vi "ASIC_CONFIGURAR IABIAS.vi"(7 "Espera acceso USB":u32=10, 8 "error in":errorcluster, 9 "IBIAS VALUE":u8 max=63 step=1, 10 "IBIAS":bool, 11 "ftHandle_in":u32) -> (0 "error out":errorcluster, 3 "ftHandle_out":u32)   [LabVIEW 2019]
panel:
  out "test":u16 format="%04x"
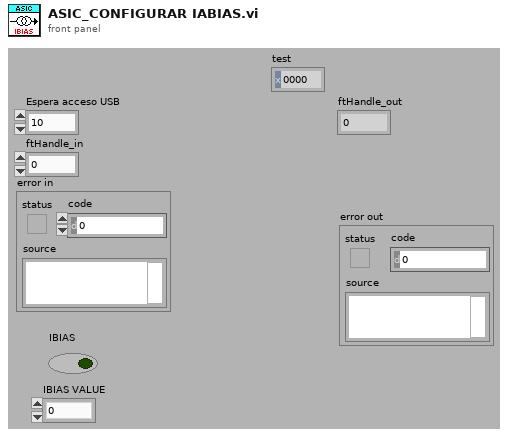
[diagram p1: front panel]
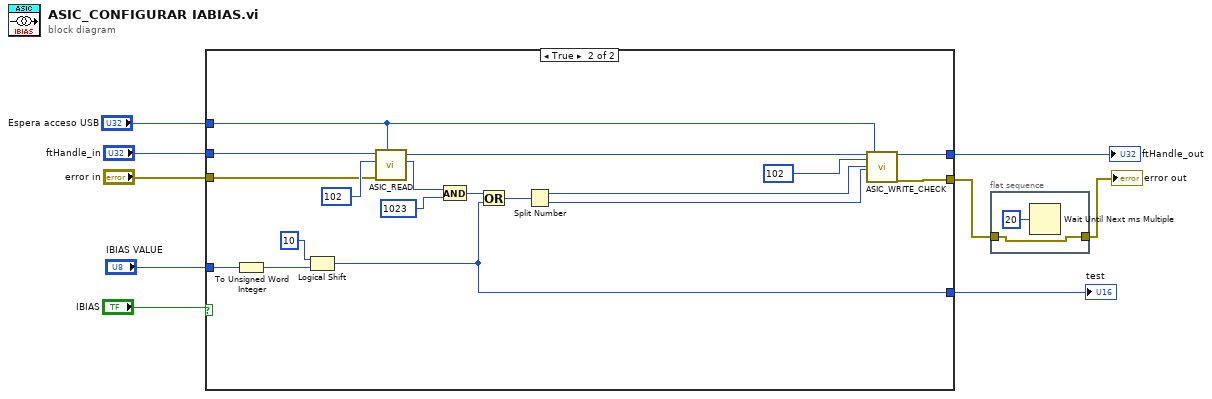
[diagram p0: block diagram]
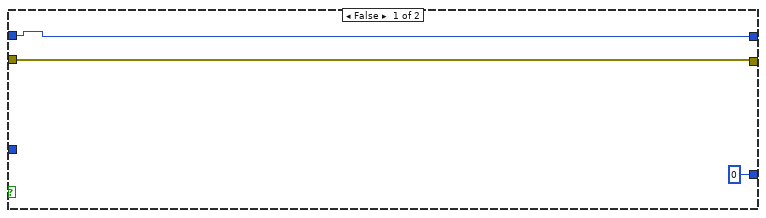
[diagram p2: hidden frame]
diagram:
  n1 = case shown="True" "IBIAS" {
    tunnel: [w10 w30] -> w9
    tunnel: [w12 w29] -> w2
    tunnel: "ftHandle_in" -> [w10 w26]
    tunnel: "error in" -> [w12 w25]
    tunnel: "Espera acceso USB" -> [_ w24]
    tunnel: [u16 0 w15] -> w5
    tunnel: "IBIAS VALUE" -> [_ w14]
    frame False {
    }
    frame True {
      n2 = To Unsigned Word Integer(number=w14) -> (unsigned 16bit integer=w13:u16)
      n3 = Logical Shift(y=u16 10 ("x"), x=w13) -> (x << y=w15:u16)
      n4 = call "ASIC_READ.vi"("Espera acceso USB"=w24, "error in"=w25, "Direccion Registro Asic"=u8 102, "ftHandle_in"=w26) -> ("Valor Asic"=w20:u16, "ftHandle_out"=w23:u32)  [unwired: 5 in, 1 out]
      n5 = And(x=w20, y=u16 1023) -> (x .and. y?=w18:u16)
      n6 = Or(x=w18, y=w15) -> (x .or. y?=w17:u16)
      n7 = Split Number(x=w17) -> (hi(x)=w22:u8, lo(x)=w21:u8)
      n8 = call "ASIC_WRITE_CHECK.vi"("ftHandle_in"=w23, "Direccion Registro Asic"=u8 102, "Byte Alto"=w22, "Byte Bajo"=w21, "Espera acceso USB 2"=w24) -> ("ftHandle_out"=w30:u32, "error out"=w29:errorcluster)  [unwired: 12 in, 1 out]
    }
  }
  "ftHandle_out" <- w9
  "test" <- w5
  n9 = flat-sequence {
    tunnel: w2 -> [w31]
    tunnel: [w31] -> w1
    frame #0 {
      n10 = Wait Until Next ms Multiple(millisecond multiple=u32 20) -> ()  [unwired: 1 out]
    }
  }
  "error out" <- w1
